vi "wind speed final.vi"(8 "error in (no error)":errorcluster, 10 "LINX Resource":T1, 11 "Numeric 3":dbl) -> (2 "Numeric 2":dbl, 3 "Numeric 4":dbl)   [LabVIEW 2020]
uses:
  <vilib>/MakerHub/LINX/Private/Type Defs/LINX Ref.ctl
  <vilib>/MakerHub/LINX/Private/Type Defs/Platform.ctl
  <vilib>/MakerHub/LINX/Private/Type Defs/Interface.ctl
  <vilib>/MakerHub/LINX/Private/Device/Type Defs/LINX Device Config.ctl
  <vilib>/MakerHub/LINX/Private/Device/Type Defs/TCP Config.ctl
  <vilib>/MakerHub/LINX/Private/Device/Type Defs/Channels.ctl
  <vilib>/MakerHub/LINX/Public/Peripherals/Digital/Digital Read 1 Chan.vi
  <vilib>/MakerHub/LINX/Public/Peripherals/Digital/Digital Read N Chans.vi
  <vilib>/MakerHub/LINX/Private/Local IO/LinxDigitalRead.vi
  <vilib>/MakerHub/LINX/Public/Utilities/Check Channel.vi
  <vilib>/MakerHub/LINX/Private/Utilties/Generate Error.vi
  <vilib>/MakerHub/LINX/LMH-LINX.lvlib
  <vilib>/MakerHub/LINX/Private/Device/Device.lvlib
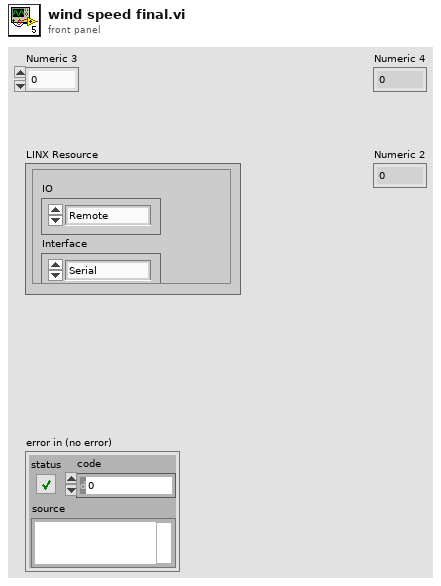
[diagram p1: front panel]
types:
  T1 = typedef "LMH-LINX.lvlib/LINX Ref.ctl" = cluster{"IO":T2, "Interface":T3, "LINX Device Config":T4}
  T2 = typedef "LMH-LINX.lvlib/Platform.ctl" = enum16{"Remote", "Local"}
  T3 = typedef "LMH-LINX.lvlib/Interface.ctl" = enum16{"Serial", "TCP"}
  T4 = typedef "LMH-LINX.lvlib/Device.lvlib/LINX Device Config.ctl" = cluster{"Interface":T3, "COM Port":refnum<visa-resource-name>, "TCP Configuration":T5, "Device Family":u8, "Device ID":u8, "Device Name":string, "TCP Ref":refnum<k5>, "Channels":T6}
  T5 = typedef "LMH-LINX.lvlib/Device.lvlib/TCP Config.ctl" = cluster{"IP Address":string, "Port":u16}
  T6 = typedef "LMH-LINX.lvlib/Channels.ctl" = cluster{"DI":u8[], "DO":u8[], "AI":u8[], "AO":u8[], "PWM":u8[], "QE":u8[], "UART":u8[], "I2C 2":u8[], "SPI":u8[], "CAN":u8[], "Servo":u8[], "AI Ref (V)":dbl, "AI Resolution (Bits)":u8, "AO Ref (V)":dbl, "AO Resolution (Bits)":u8}
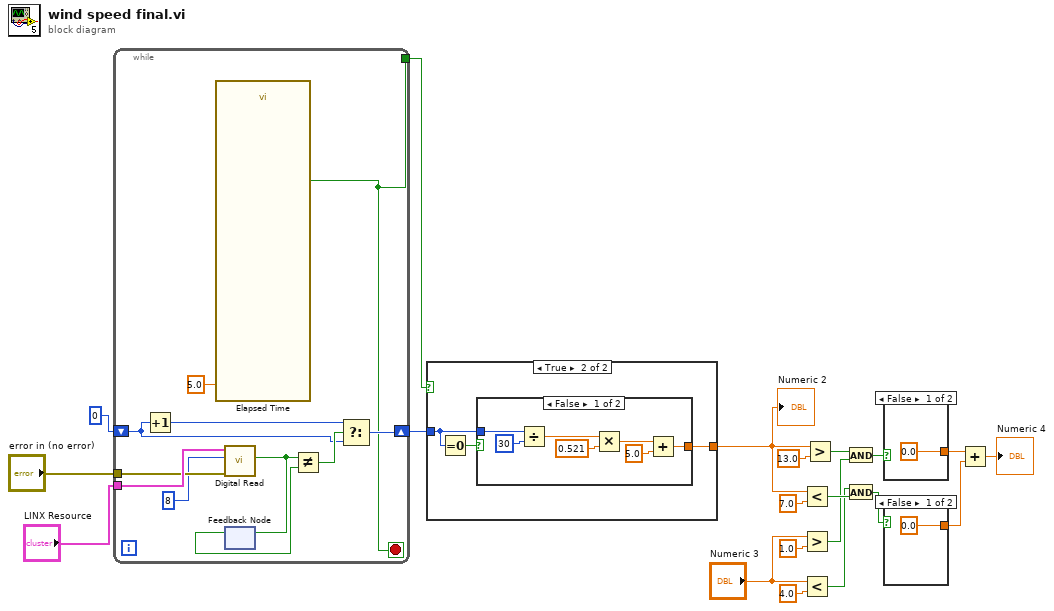
[diagram p0: block diagram]
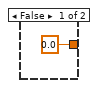
[diagram p2: hidden frame]
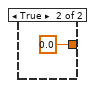
[diagram p3: hidden frame]
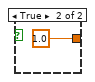
[diagram p4: hidden frame]
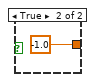
[diagram p5: hidden frame]
diagram:
  n1 = while {
    tunnel: "LINX Resource" -> [w31]
    tunnel: "error in (no error)" -> [w30]
    shift-right: [w22] -> w19
    shift-left: 0 ("Numeric in") -> [w23]
    tunnel: [w21] -> w20
    stop <- w21 stop-if-true
    n2 = Increment(x=w23) -> (x+1=w28:i32)
    n3 = call "Elapsed Time"("Time Target (s)"=5.0) -> ("Time has Elapsed"=w21:bool)  [unwired: 11 in, 7 out]
    n4 = call-poly <vilib>:"Digital Read.vi"("Error In"=w30, "DI Channel"=u8 8, "LINX Resource"=w31) -> ("DI Value"=w25:bool)  [unwired: 6 in, 2 out]
    n5 = feedback #1() -> (w26:bool)  [unwired: 1 in]
    n6 = feedback-in #1(w25) -> ()
    n7 = Not Equal?(x=w25, y=w26) -> (x != y?=w24:bool)
    n8 = Select(t=w28, s=w24, f=w23) -> (s? t:f=w22:i32)
  }
  n9 = case shown="True" w20 {
    tunnel: w19 -> [_ w33]
    tunnel: [0.0 w35] -> w5
    frame False {
    }
    frame True {
      n10 = Equal To 0?(x=w33) -> (x = 0?=w34:bool)
      n11 = case shown="False" w34 {
        tunnel: [w40 0.0] -> w35
        tunnel: w33 -> [w42 _]
        frame False {
          n12 = Divide(x=w42, y=30) -> (x/y=w41:dbl)
          n13 = Multiply(x=w41, y=0.521) -> (x*y=w39:dbl)
          n14 = Add(x=w39, y=5.0) -> (x+y=w40:dbl)
        }
        frame True {
        }
      }
    }
  }
  "Numeric 2" <- w5
  n15 = Less?(x=w5, y=7.0) -> (x < y?=w9:bool)
  n16 = Greater?(x="Numeric 3", y=1.0) -> (0:w7:bool)
  n17 = Less?(x="Numeric 3", y=4.0) -> (x < y?=w8:bool)
  n18 = Greater?(x=w5, y=13.0) -> (0:w6:bool)
  n19 = And(x=w6, y=w7) -> (x .and. y?=w13:bool)
  n20 = And(x=w8, y=w9) -> (x .and. y?=w10:bool)
  n21 = case shown="False" w13 {
    tunnel: [0.0 -1.0] -> w11
    frame False {
    }
    frame True {
    }
  }
  n22 = case shown="False" w10 {
    tunnel: [0.0 1.0] -> w12
    frame False {
    }
    frame True {
    }
  }
  n23 = Add(x=w11, y=w12) -> (x+y=→"Numeric 4":dbl)
